vi "Create PV Data.vi"(8 "error in":errorcluster, 11 "Base Interface in":refnum<class "Base Interface.lvclass">) -> (0 "error out":errorcluster, 2 "PV data out":refnum<class "PV Data.lvclass">, 3 "Base Interface out":refnum<class "Base Interface.lvclass">)   [LabVIEW 2020, in "PV Access.lvlib" / "PV Data.lvlib" / "Base Interface.lvclass"]
uses:
  Base Interface.lvclass
  PV Data/PV Data.lvclass
  Type Definition/Type Definition.lvclass
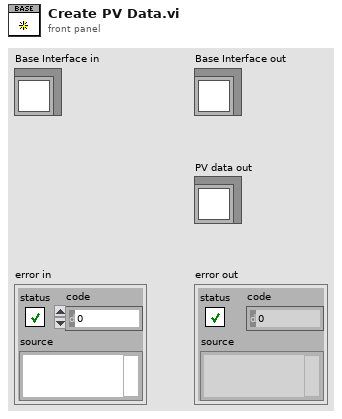
[diagram p1: front panel]
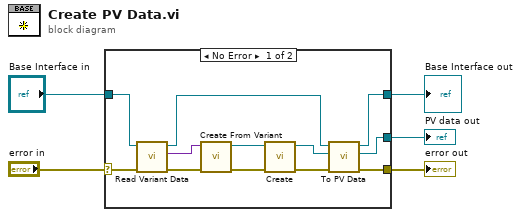
[diagram p0: block diagram]
diagram:
  n1 = case shown="No Error" "error in" {
    selector: "error in" -> [w10 w19]
    tunnel: "Base Interface in" -> [w8 w18]
    tunnel: [w14 w19] -> w3
    tunnel: [w11 w18] -> w1
    tunnel: [w12 _] -> w2
    frame No Error {
      n2 = call-dynamic "Read Variant Data.vi"("error in"=w10, "Base Interface in"=w8) -> ("error out"=w9:errorcluster, "data"=w6:variant, "Base Interface out"=w7:refnum<class "Base Interface.lvclass">)  [unwired: 7 in]
      n3 = call "Create From Variant.vi"("error in (no error)"=w9, "value"=w6) -> ("error out"=w17:errorcluster, "Type Definition out"=w16:refnum<class "Type Definition.lvclass">)  [unwired: 7 in, 1 out]
      n4 = call "Create.vi"("error in"=w17, "Type Definition"=w16) -> ("error out"=w15:errorcluster, "PV Data"=w13:refnum<class "PV Data.lvclass">)  [unwired: 8 in]
      n5 = call-dynamic "To PV Data.vi"("error in"=w15, "PV data in"=w13, "Base Interface in"=w7) -> ("error out"=w14:errorcluster, "PV data out"=w12:refnum<class "PV Data.lvclass">, "Base Interface out"=w11:refnum<class "Base Interface.lvclass">)  [unwired: 6 in]
    }
    frame Error {
    }
  }
  "error out" <- w3
  "Base Interface out" <- w1
  "PV data out" <- w2
